vi "PrepareIndividualPorts.vi"(0 "Target Ports":i32[](array[numeric])=[61540, 61542, 61544, 61546]) -> (1 "Connection IDs":refnum<k16>[](array[refnum]), 3 "Error(s) Out":errorcluster[](array[cluster]))   [LabVIEW 2012]
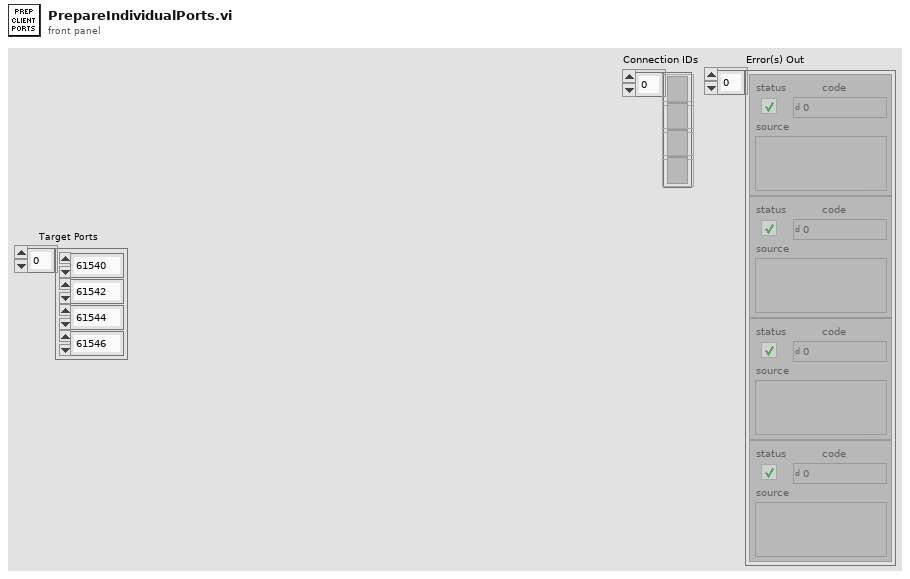
[diagram p1: front panel]
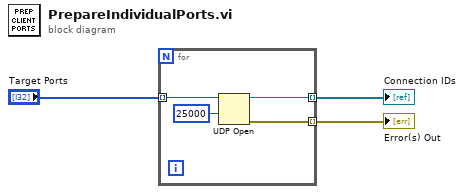
[diagram p0: block diagram]
diagram:
  n1 = for {
    tunnel: "Target Ports" -> [w7] mode=indexing
    tunnel: [w5] -> w2 mode=indexing
    tunnel: [w4] -> w1 mode=indexing
    n2 = UDP Open(9:25000 ("timeout ms (25000)"), 11:w7) -> (port=w5:refnum<k16>, 0:w4:errorcluster)  [unwired: 3 in, 1 out]
  }
  "Connection IDs" <- w2
  "Error(s) Out" <- w1
